vi "subPatternMatch.vi"(0 "Image In":T2, 1 "error in":errorcluster, 2 "Template File Path (Pattern Matching 1)":path[](array[path]), 3 "Parameters (Pattern Matching 1)":T1={"Number of Matches Requested"=1, "Minimum Match Score"=450.0, "Angle Ranges"=[{"Start Angle"=-10.0, "End Angle"=10.0}]}, 4 "index":i32) -> (20 "Image Out":T2, 21 "error out":errorcluster, 23 "Calibrated Matches (Pattern Matching 1)":T3(array[cluster]) {"Bounding Box"."y" format="%.2f"; "Bounding Box"."x" format="%.2f"; "Position"."y" format="%.2f"; "Position"."x" format="%.2f"; "Score" format="%.2f"; "Scale" format="%.2f"; "Angle" format="%.2f"}, 24 "Number of Matches (Pattern Matching 1)":i32)   [LabVIEW 2017]
doc: "Creates, edits, and runs vision algorithms using NI Vision Assistant.\n\nWhen you place this Express VI on the block diagram, NI Vision Assistant launches. Create an algorithm using the Vision Assistant processing functions. After you create an algorithm, you can select the controls and indicators that you want to be able to programmatically set in LabVIEW. Double-click the Vision Assistant Express VI to edit the algorithm."
uses:
  <vilib>/vision/Image Controls.llb/IMAQ Image.ctl
  <vilib>/vision/NI_Vision_Development_Module.lvlib
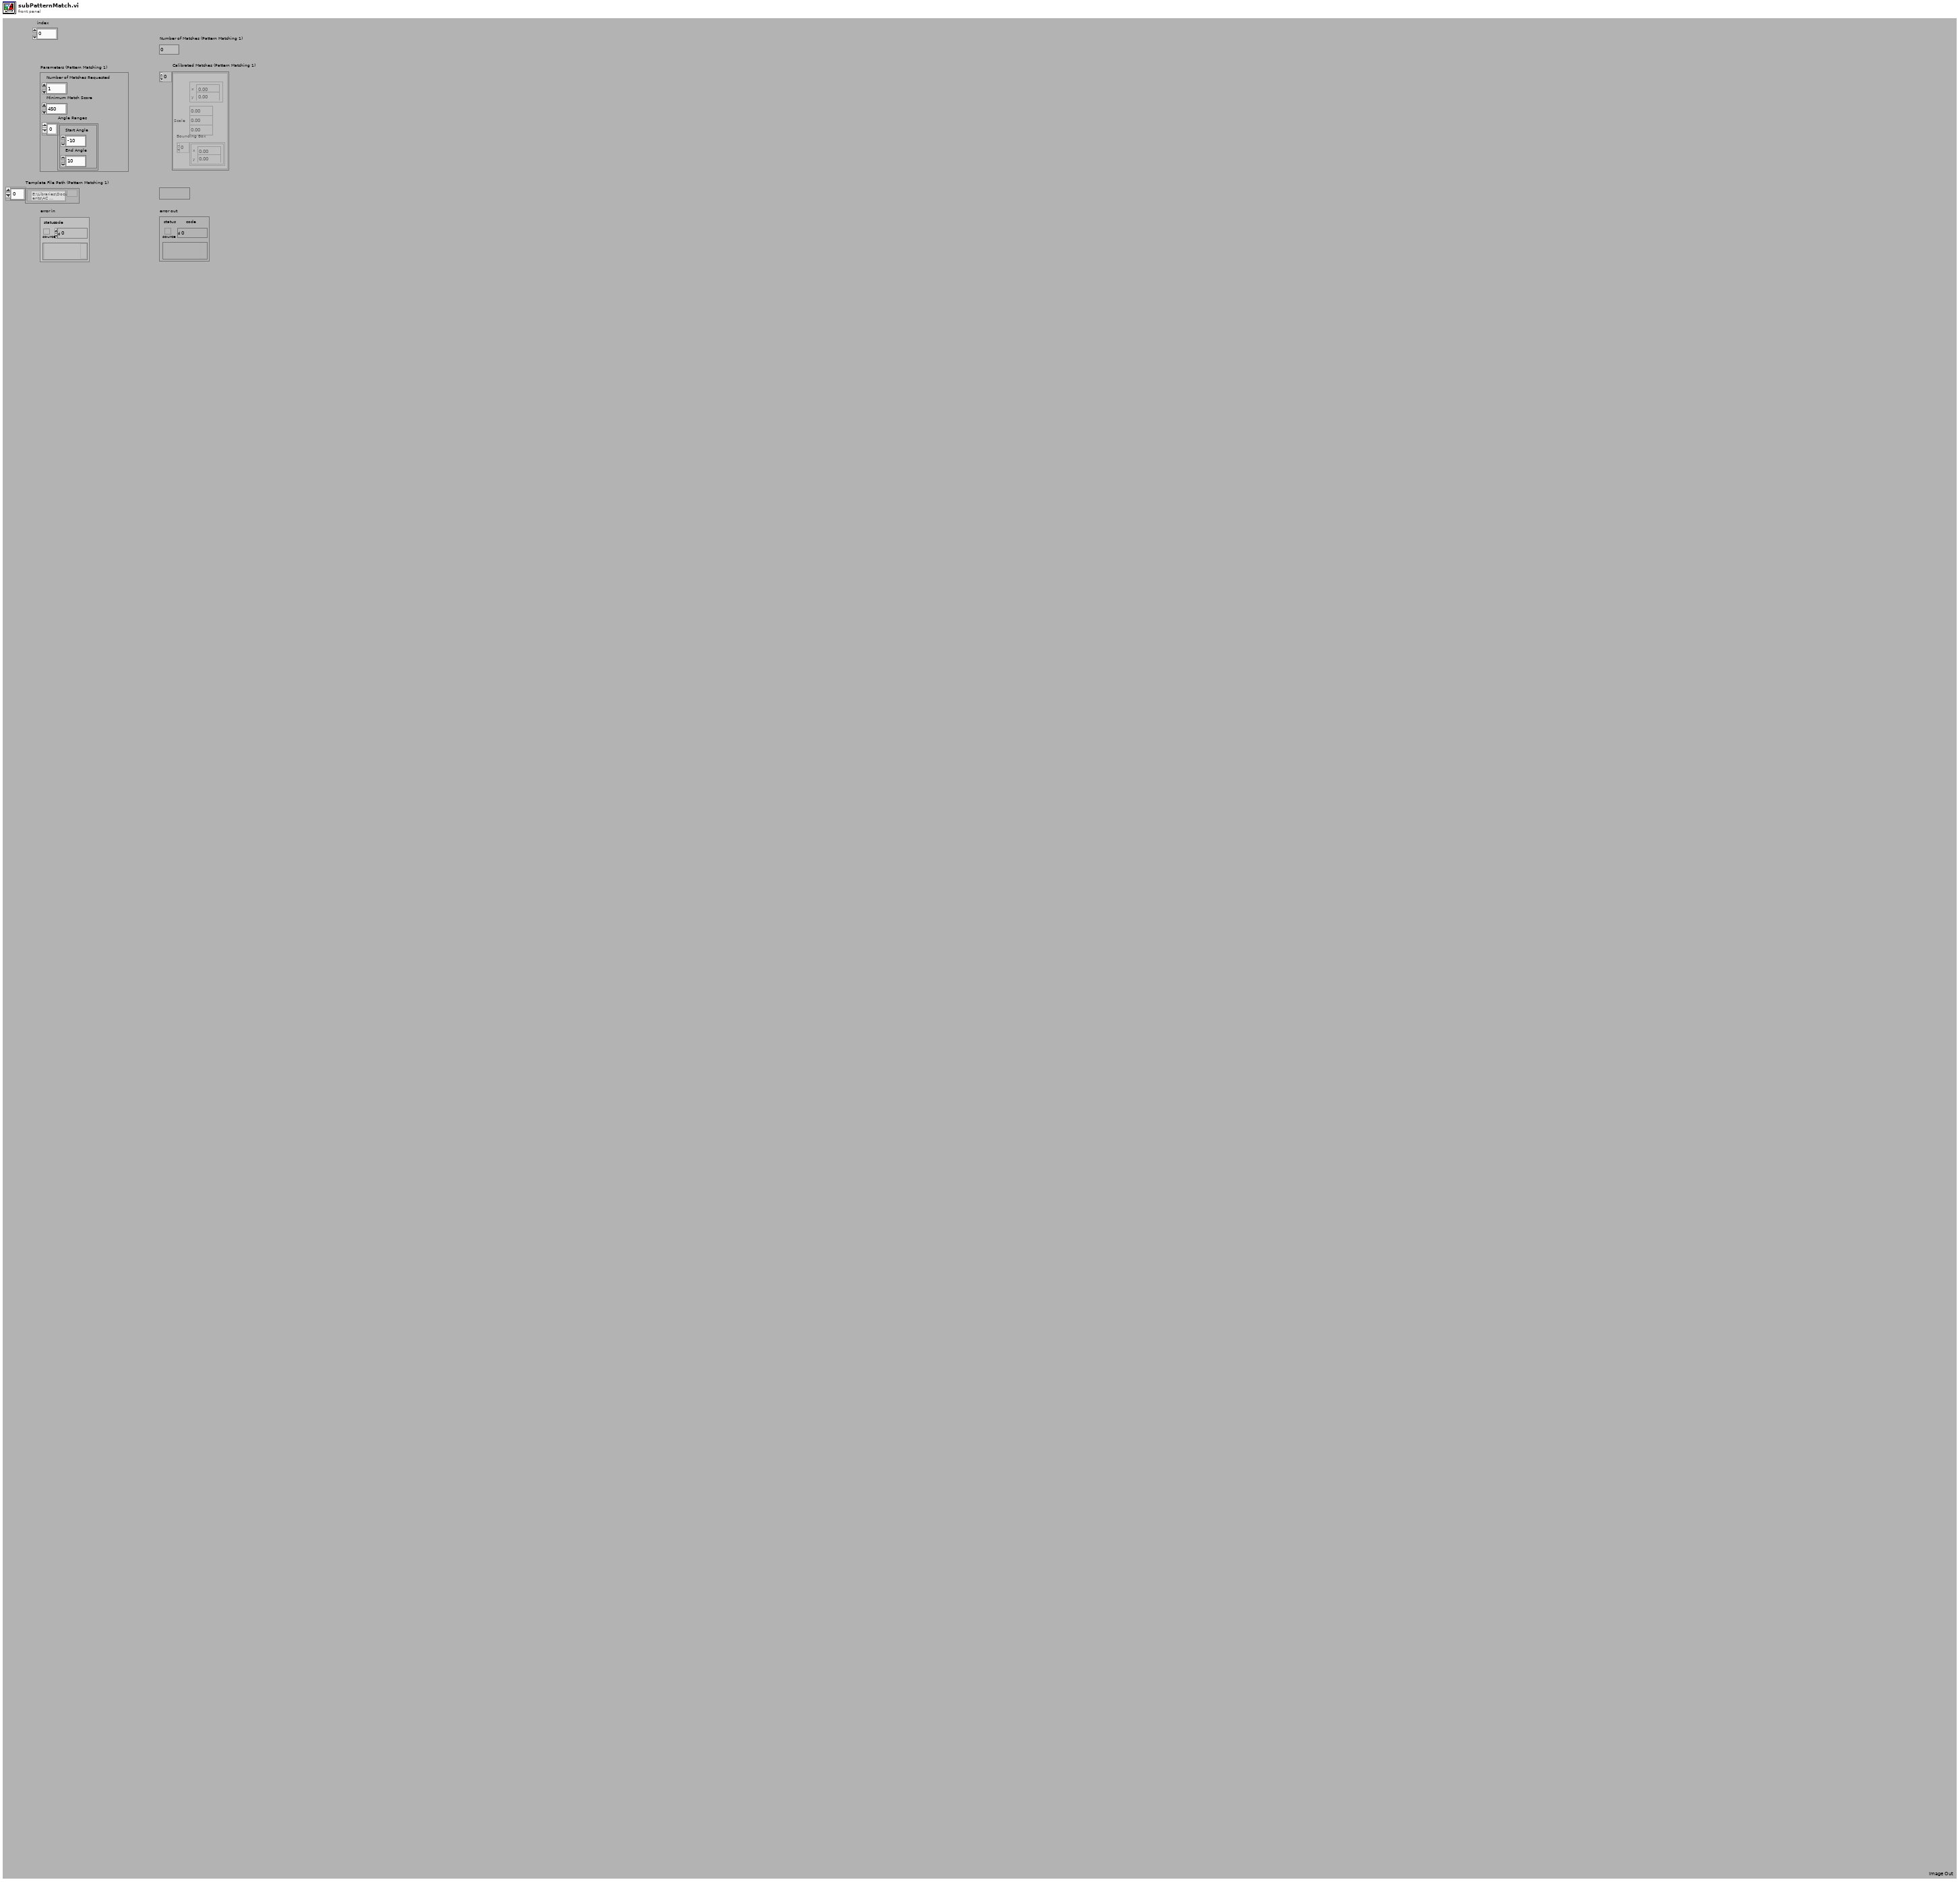
[diagram p1: front panel]
types:
  T1 = cluster{"Number of Matches Requested":i32, "Minimum Match Score":sgl, "Angle Ranges":cluster{"Start Angle":sgl, "End Angle":sgl}[]}
  T2 = typedef "IMAQ Image.ctl" = refnum<image>
  T3 = cluster{"Position":cluster{"x":sgl, "y":sgl}, "Angle":sgl, "Scale":sgl, "Score":sgl, "Bounding Box":cluster{"x":sgl, "y":sgl}[]}[]
  T4 = cluster{"Global Rectangle":i32[], "Contours":cluster{"ID":enum32{"External", "Internal"}, "Type":u32, "Coordinates":i32[]}[]}
  T5 = typedef "Image Type" = u32
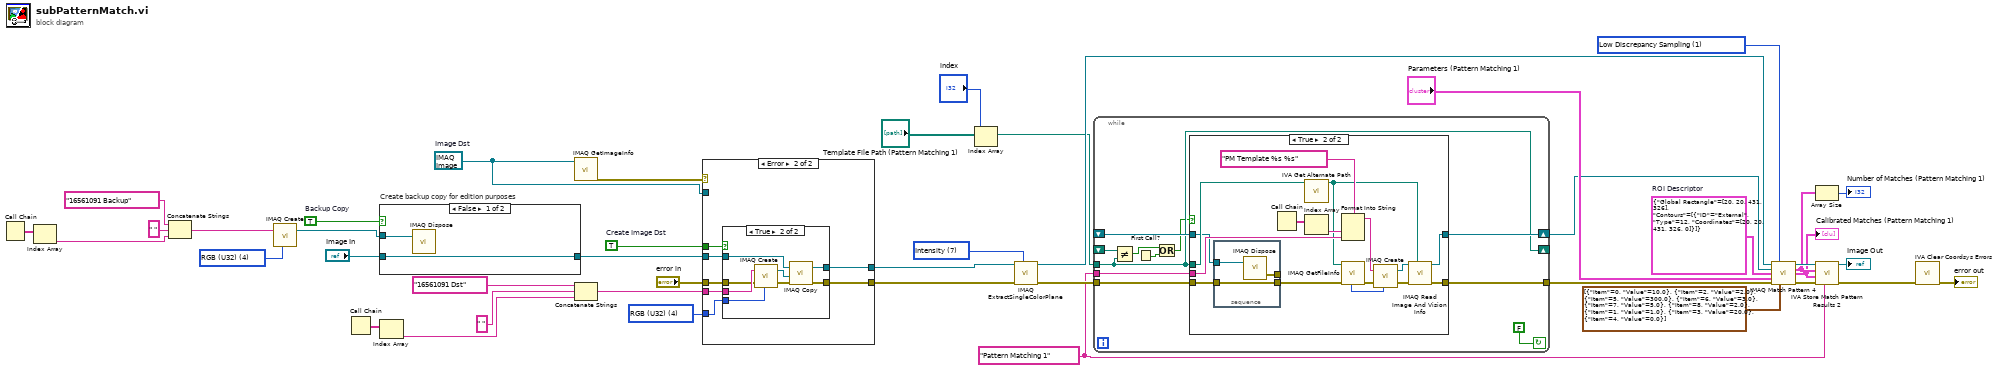
[diagram p0: block diagram]
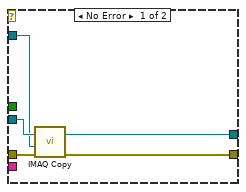
[diagram p3: hidden frame]
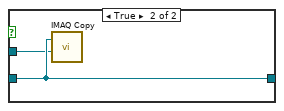
[diagram p5: hidden frame]
diagram:
  w15 = 1 items=["All", "Low Discrepancy Sampling", "Grayscale Value Pyramid", "Gradients Pyramid"] ("Algorithm")
  w11 = "Pattern Matching 1" ("Step Name")
  w14 = T4 {"Global Rectangle"=[20, 20, 431, 326], "Contours"=[{"ID"=enum."External", "Type"=12, "Coordinates"=[20, 20, 431, 326, 0]}]}  # ROI Descriptor
  w23 = 7 items=["Red", "Green", "Blue", "Hue", "Saturation", "Luminance", "Value", "Intensity"] ("Color Plane")
  w24 = T5 4 items=["Grayscale (U8)", "Grayscale (I16)", "Grayscale (SGL)", "Complex (CSG)", "RGB (U32)", "HSL (U32)", "RGB (U64)", "Grayscale (U16)"] ("Image Dst Type")
  w25 = T5 4 items=["Grayscale (U8)", "Grayscale (I16)", "Grayscale (SGL)", "Complex (CSG)", "RGB (U32)", "HSL (U32)", "RGB (U64)", "Grayscale (U16)"] ("Image Type")
  w43 = TRUE  # Backup Copy
  w42 = T2 refnum  # Image Dst
  w37 = TRUE  # Create Image Dst
  n1 = Call Chain() -> (call chain=w31:string[])
  n2 = Index Array(array=w31) -> (element=w30:string)  [unwired: 1 in]
  n3 = Concatenate Strings("16561091 Backup" ("Backup Image Name"), " ", w30) -> (w27:string)
  n4 = call "IMAQ Create"("Image Name"=w27, "Image Type"=w25) -> ("New Image"=w26:T2)  [unwired: 2 in, 2 out]
  n5 = Call Chain() -> (call chain=w36:string[])
  n6 = case "Create backup copy for edition purposes" shown="False" w43 {
    tunnel: [w45 w47] -> w39
    tunnel: "Image In" -> [w45 w47]
    tunnel: w26 -> [w44 w46]
    frame False {
      n7 = call "IMAQ Dispose"("Image"=w44) -> ()  [unwired: 2 in, 4 out]
    }
    frame True {
      n8 = call "IMAQ Copy"("Image Dst"=w46, "Image Src"=w47) -> ()  [unwired: 1 in, 5 out]
    }
  }
  n9 = Index Array(array=w36) -> (element=w34:string)  [unwired: 1 in]
  n10 = call "IMAQ GetImageInfo"("Image"=w42) -> ("error out"=w41:errorcluster)  [unwired: 1 in, 9 out]
  n11 = Concatenate Strings("16561091 Dst" ("Image Dst Name"), " ", w34) -> (w32:string)
  n12 = case shown="Error" w41 {
    tunnel: [w52 w56] -> w22
    tunnel: [w51 w55] -> w21
    tunnel: w39 -> [w50 w57]
    tunnel: "error in" -> [w49 w53]
    tunnel: w42 -> [w48 _]
    tunnel: w32 -> [_ w59]
    tunnel: w24 -> [_ w58]
    tunnel: w37 -> [_ w54]
    frame No Error {
      n13 = call "IMAQ Copy"("error in (no error)"=w49, "Image Dst"=w48, "Image Src"=w50) -> ("error out"=w51:errorcluster, "Image Dst Out"=w52:T2)  [unwired: 3 out]
    }
    frame Error {
      n14 = case shown="True" w54 {
        tunnel: w59 -> [_ w69]
        tunnel: w58 -> [_ w68]
        tunnel: w57 -> [w61 w66]
        tunnel: [w61 w65] -> w56
        tunnel: [w60 w64] -> w55
        tunnel: w53 -> [w60 w62]
        frame False {
        }
        frame True {
          n15 = call "IMAQ Create"("Image Name"=w69, "Image Type"=w68, "error in (no error)"=w62) -> ("New Image"=w67:T2, "error out"=w63:errorcluster)  [unwired: 1 in, 1 out]
          n16 = call "IMAQ Copy"("error in (no error)"=w63, "Image Dst"=w67, "Image Src"=w66) -> ("error out"=w64:errorcluster, "Image Dst Out"=w65:T2)  [unwired: 3 out]
        }
      }
    }
  }
  n17 = Index Array(array="Template File Path (Pattern Matching 1)", index="index") -> (element=w2:path)
  n18 = call "IMAQ ExtractSingleColorPlane"("Color Plane"=w23, "error in (no error)"=w21, "Image Src"=w22) -> ("error out"=w16:errorcluster, "Image Dst Out"=w19:T2)  [unwired: 1 in, 6 out]
  n19 = while {
    shift-right: [w80] -> w8
    shift-left: _ -> [w79]
    tunnel: [w77] -> w7
    tunnel: w16 -> [w76]
    tunnel: w2 -> [w73]
    tunnel: w11 -> [w75]
    shift-right: [w73] -> _
    shift-left: _ -> [w74]
    stop <- FALSE continue-if-true
    n20 = Not Equal?(x=w74, y=w73) -> (x != y?=w71:bool)
    n21 = First Call?() -> (First Call?: T/F=w72:bool)
    n22 = Or(x=w71, y=w72) -> (x .or. y?=w70:bool)
    n23 = case shown="True" w70 {
      tunnel: [w82 w96] -> w80
      tunnel: w79 -> [w82 w88]
      tunnel: [w81 w93] -> w77
      tunnel: w76 -> [w81 w87]
      tunnel: w73 -> [_ w89]
      tunnel: w75 -> [_ w90]
      frame False {
      }
      frame True {
        n24 = stacked-sequence {
          tunnel: w88 -> [w101]
          tunnel: w87 -> [w100]
          tunnel: [w100] -> w83
          tunnel: [w99] -> _
          frame #0 {
            n25 = call "IMAQ Dispose"("Image"=w101) -> ("error out"=w99:errorcluster)  [unwired: 2 in, 3 out]
          }
        }
        n26 = Call Chain() -> (call chain=w92:string[])
        n27 = call <vilib>:"IVA Get Alternate Path.vi"("Path In"=w89) -> ("Path Out"=w85:path)  [unwired: 10 out]
        n28 = Index Array(array=w92) -> (element=w91:string)  [unwired: 1 in]
        n29 = Format Into String(format string="PM Template %s %s" ("Image Name"), w91, w90) -> (resulting string=w98:string)  [unwired: 2 in, 1 out]
        n30 = call "IMAQ GetFileInfo"("error in (no error)"=w83, "File Path"=w85) -> ("error out"=w84:errorcluster, "Image Type"=w86:T5)  [unwired: 3 in, 5 out]
        n31 = call "IMAQ Create"("Image Name"=w98, "Image Type"=w86, "error in (no error)"=w84) -> ("New Image"=w95:T2, "error out"=w94:errorcluster)  [unwired: 1 in, 1 out]
        n32 = call "IMAQ Read Image And Vision Info"("File Path"=w85, "error in (no error)"=w94, "Image"=w95) -> ("error out"=w93:errorcluster, "Image Out"=w96:T2)  [unwired: 1 in, 6 out]
      }
    }
  }
  n33 = call "IMAQ Match Pattern 4"("Image"=w19, "Algorithm"=w15, "Template Image"=w8, "ROI Descriptor"=w14, "Parameters"="Parameters (Pattern Matching 1)", "error in (no error)"=w7, "Advanced Options"=cluster{"Item":u16, "Value":dbl}[] [{"Item"=0, "Value"=10.0}, {"Item"=2, "Value"=2.0}, {"Item"=5, "Value"=300.0}, {"Item"=6, "Value"=3.0}, {"Item"=7, "Value"=5.0}, {"Item"=8, "Value"=2.0}, {"Item"=1, "Value"=1.0}, {"Item"=3, "Value"=20.0}, {"Item"=4, "Value"=0.0}]) -> ("Image (duplicate)"=w17:T2, "Matches (pixel)"=w10:T3, "Matches (real-world)"=w9:T3, "error out"=w18:errorcluster)  [unwired: 4 in, 1 out]
  "Calibrated Matches (Pattern Matching 1)" <- w9
  n34 = Array Size(array=w10) -> (size(s)=→"Number of Matches (Pattern Matching 1)":i32)
  n35 = call <vilib>:"IVA Store Match Pattern Results 2.vi"("Step Name"=w11, "error in (no error)"=w18, "Matches (real-world)"=w9, "Matches (pixel)"=w10, "Image in"=w17) -> ("error out"=w6:errorcluster, "Image dup"=→"Image Out":T2)  [unwired: 1 in, 4 out]
  n36 = call <vilib>:"IVA Clear Coordsys Errors.vi"("error in (no error)"=w6) -> ("error out"=→"error out":errorcluster)  [unwired: 10 in]
